vi "nx-100 (FPGA).vi"() -> ()   [LabVIEW 2019]
uses:
  <vilib>/Platform/TimedLoop/XDataNode/wakeup.ctl
  <vilib>/Platform/TimedLoop/XDataNode/XDNodeRunTimeDep.lvlib
  <vilib>/Platform/TimedLoop/XDataNode/nitl_modes.ctl
  <vilib>/Platform/TimedLoop/XDataNode/timing_clust.ctl
  <vilib>/Platform/TimedLoop/XDataNode/XDataNode.xnode
  <userlib>/_NI SPI IP/FPGA/Controllers/Public/Spi Master Inputs.ctl
  <vilib>/eio/EIONode/EIONode.xnode
  <vilib>/rvi/eio/common/nirviEmuTemplateMethod_errors.vi
  <vilib>/eio/EIOMethodNode/EIOMethodNode.xnode
  Controls/SPI Channels.ctl
  <vilib>/rvi/DataTransferAndStorage/Container/XNode/niFpgaContainer.xnode
  <vilib>/rvi/FIFO/Fifo_Resource/niFpgaFifoEmulationRefIn.vi
  <userlib>/_NI SPI IP/FPGA/Controllers/Public/Transfer Settings.ctl
  <vilib>/rvi/interface/RandomDataEmulation/nirviRandomDataFpgaReadWriteTemplate.vi
panel:
  in  "LCD Lt Timeout":i32=10000
  in  "Average?":bool
  out "Averaged Data":u16[](array[numeric])
  in  "N (# of Ave Pts 32 max)":i16
  in  "Onboard AO SPI Settings":T1={"Divide Value"=10, "Transfer Length (bits)"=32, "CS Asserted Polarity"=FALSE, "Clock Polarity (CPOL)"=TRUE, "Clock Phase (CPHA)"=FALSE, "Lengthen MISO Setup"=TRUE, "Direction Change Bit"=0, "MOSI Starts as Output"=FALSE, "Tristatable MOSI"=FALSE} {"Direction Change Bit" max=64 step=1; "Transfer Length (bits)" min=1 max=64 step=1}
  in  "Onboard AO Setpoints":fxp<+,16,3>[](array[numeric])=[0.0, 0.0, 0.0, 0.0, 0.0, 0.0, 0.0, 0.0]
  in  "Ignition Control":bool
  in  "Onboard AI Sample Divisor":u32
  in  "LCD On/Off":bool
  in  "Onboard AI Data In":u64 format="%.0x"
  out "Onboard AI":u16[](array[numeric])
  out "Onboard AI Data":u64 format="%.0x"
  in  "Onboard AI SPI Settings":T1 {"Direction Change Bit" max=64 step=1; "Transfer Length (bits)" min=1 max=64 step=1}
  in  "LCD SPI Settings":T1={"Divide Value"=9, "Transfer Length (bits)"=64, "CS Asserted Polarity"=FALSE, "Clock Polarity (CPOL)"=FALSE, "Clock Phase (CPHA)"=FALSE, "Lengthen MISO Setup"=FALSE, "Direction Change Bit"=0, "MOSI Starts as Output"=FALSE, "Tristatable MOSI"=FALSE} {"Direction Change Bit" max=64 step=1; "Transfer Length (bits)" min=1 max=64 step=1}
  in  "LCD Message":u16 format="%.0x"
  in  "LCD Send Message":bool
  out "LCD Ready For Input":bool
  in  "nx-100 Conversion Request":bool
  in  "nx-100 Manual":bool
  in  "nx-100 Trigger":bool=TRUE
  in  "nx-100 CS Mode":enum16{"All", "CS0", "CS1"}(ring)
  in  "nx-100 AI Divisor":u32
  in  "nx-100 SPI Settings":T1 {"Direction Change Bit" max=64 step=1; "Transfer Length (bits)" min=1 max=64 step=1}
  in  "nx-100 Data In":u64 format="%.0x"
  out "nx-100 AI Data":u16[](array[numeric])
  out "nx-100 Read Data":u64 format="%.0x"
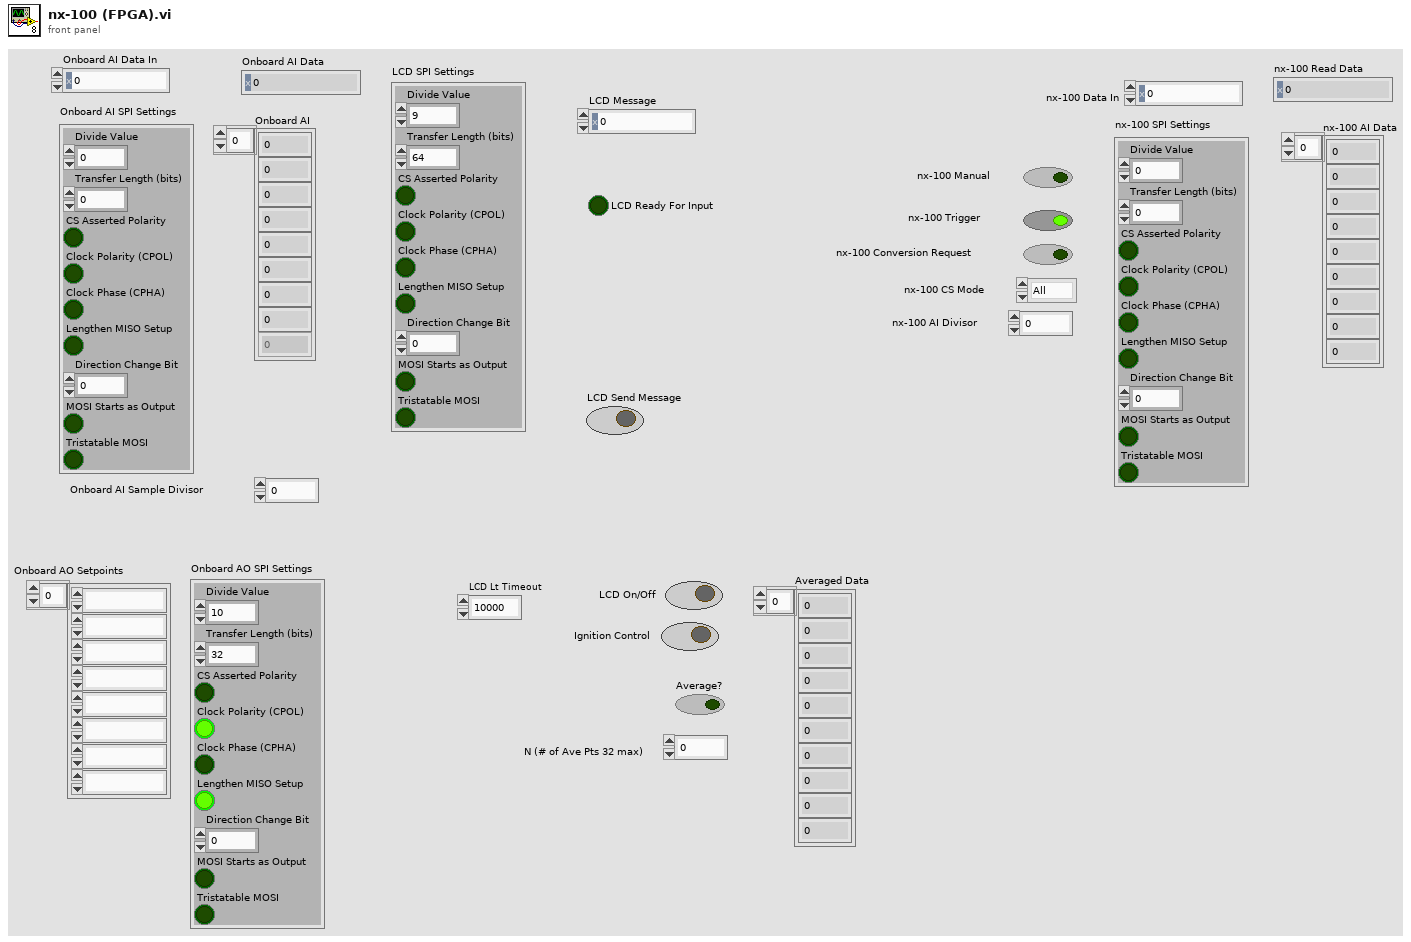
[diagram p1: front panel]
types:
  T1 = typedef "DIO SPI FPGA.lvlib/Transfer Settings.ctl" = cluster{"Divide Value":u8, "Transfer Length (bits)":u8, "CS Asserted Polarity":bool, "Clock Polarity (CPOL)":bool, "Clock Phase (CPHA)":bool, "Lengthen MISO Setup":bool, "Direction Change Bit":u8, "MOSI Starts as Output":bool, "Tristatable MOSI":bool}
  T2 = typedef "SPI Channels.ctl" = cluster{"CS":refnum<k21>, "CLK":refnum<k21>, "MOSI":refnum<k21>, "MISO":refnum<k21>}
  T3 = typedef "XDNodeRunTimeDep.lvlib/timing_clust.ctl" = cluster{"Expected End [f-1]":u64, "Actual End [f-1]":u64, "Finished Late? [f-1]":bool, "Expected End [i-1]":u64, "Actual End [i-1]":u64, "Finished Late? [i-1]":bool, "Expected Start [i]":u64, "Actual Start [i]":u64, "Expected Start [f]":u64, "Actual Start [f]":u64, "Source Name":string, "Structure Name":string, "Period":i64, "Deadline":i64, "Offset":i64, "Start":i64, "Priority":i32, "Timeout":i32, "Mode":T4, "Wakeup Reason":T5, "Error":errorcluster, "Source Type":string, "Secondary Source Type":string, "Global End Time":u64, "Global Start Time":u64, "Frame Duration":u64, "Iteration Duration":u64, "Assigned CPU":i32, "I/O Scan Engine Mode":u32}
  T4 = typedef "XDNodeRunTimeDep.lvlib/nitl_modes.ctl" = enum32{"No Change", "Process missed periods, maintain original phase", "Discard missed periods, maintain original phase", "Process missed periods, ignore original phase", "Discard missed periods, ignore original phase"}
  T5 = typedef "XDNodeRunTimeDep.lvlib/wakeup.ctl" = enum32{"Normal", "Aborted", "Asynchronous wakeup", "Timing source error", "Timed loop error", "Timeout"}
  T6 = typedef "DIO SPI FPGA.lvlib/Spi Master Inputs.ctl" = cluster{"MISO":bool}
  T7 = typedef "DIO SPI FPGA.lvlib/Spi Master Outputs.ctl" = cluster{"Chip Select":bool, "Clock":bool, "MOSI":bool, "MOSI OE":bool}
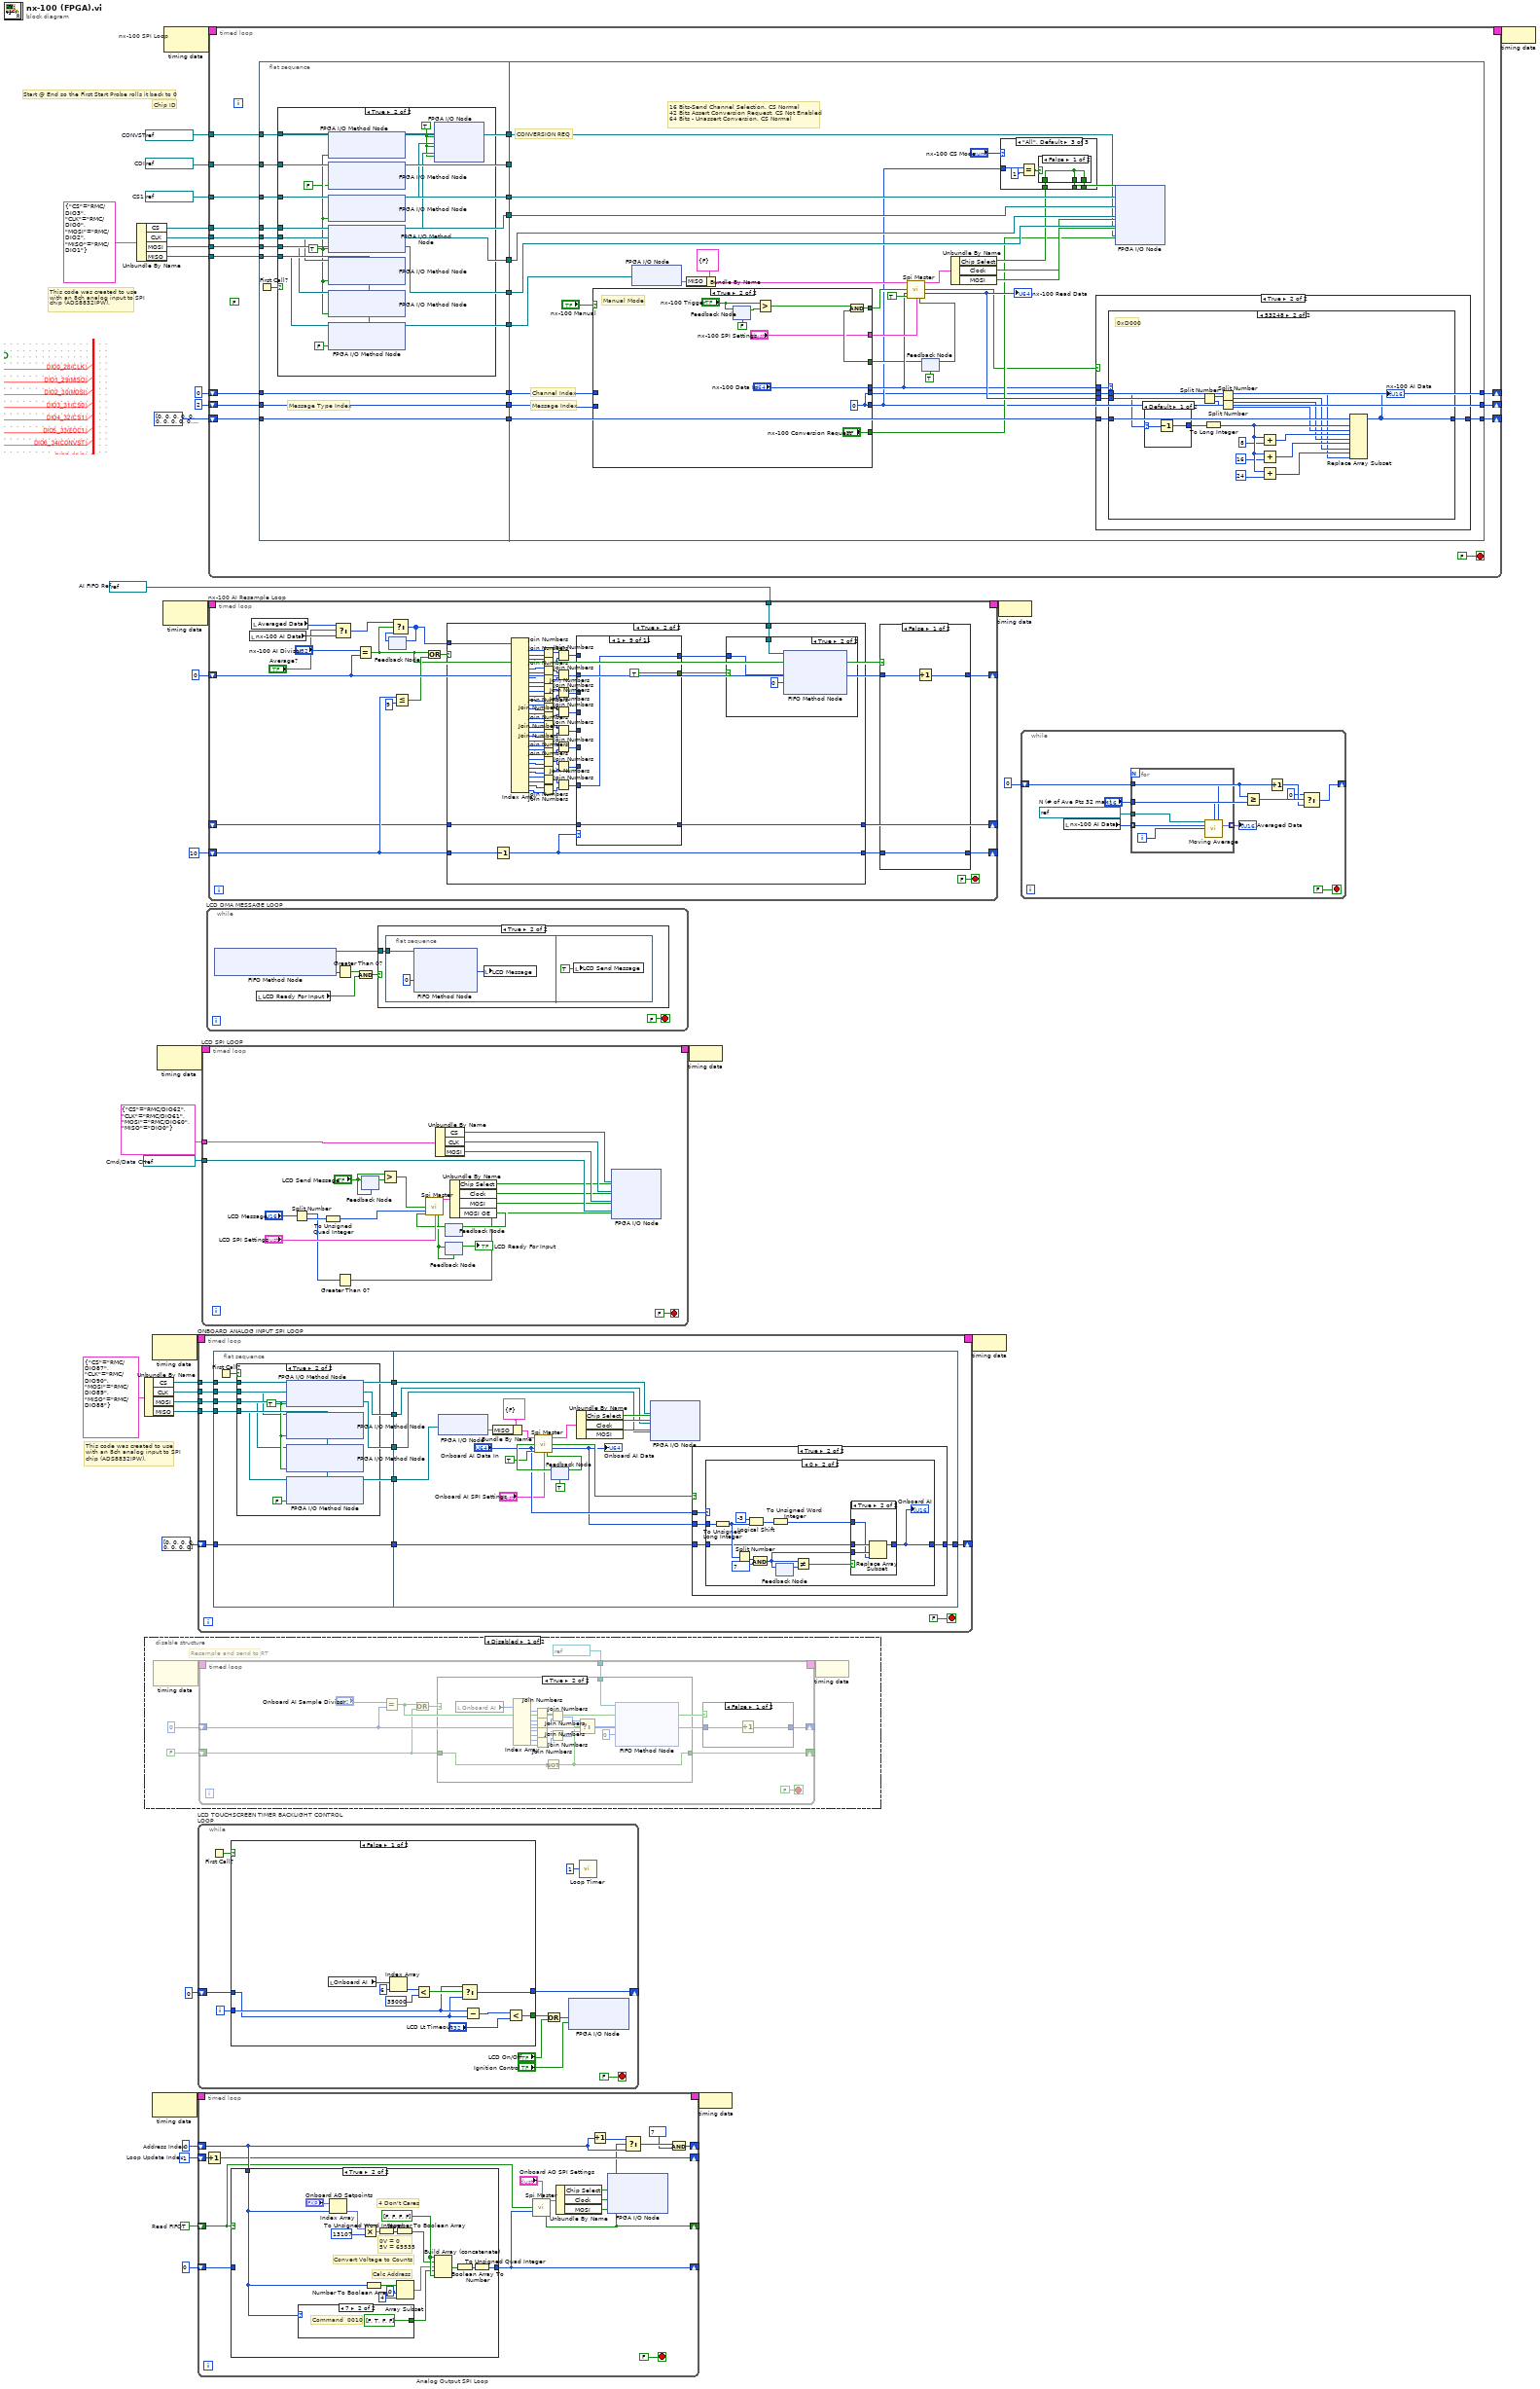
[diagram p0: block diagram]
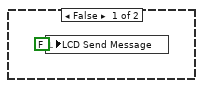
[diagram p2: hidden frame]
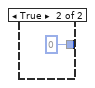
[diagram p3: hidden frame]
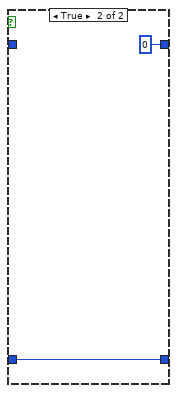
[diagram p6: hidden frame]
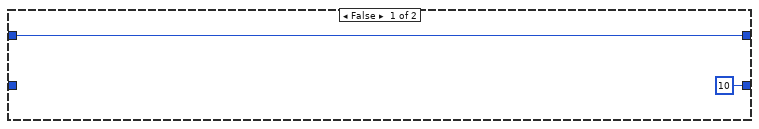
[diagram p7: hidden frame]
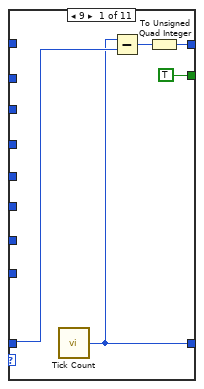
[diagram p9: hidden frame]
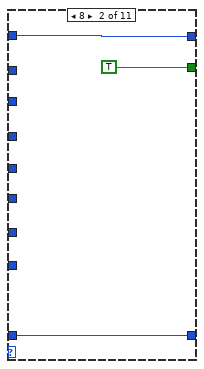
[diagram p10: hidden frame]
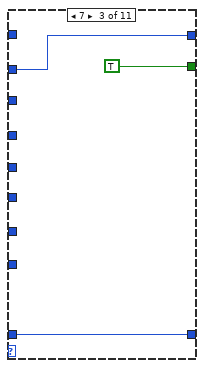
[diagram p11: hidden frame]
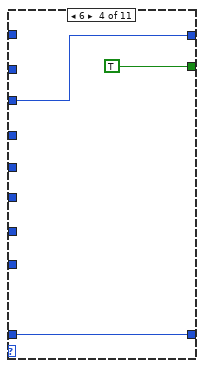
[diagram p12: hidden frame]
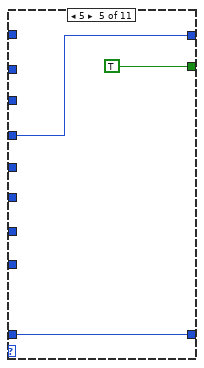
[diagram p13: hidden frame]
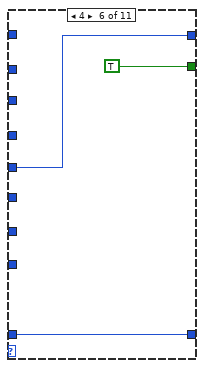
[diagram p14: hidden frame]
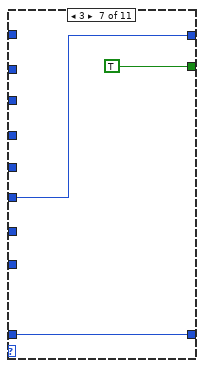
[diagram p15: hidden frame]
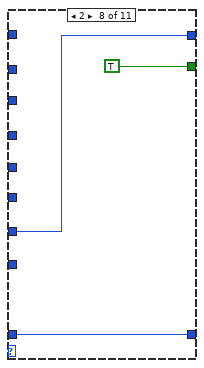
[diagram p16: hidden frame]
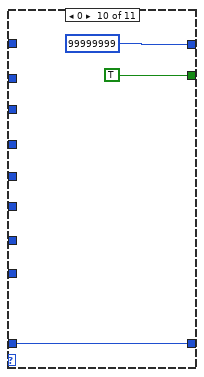
[diagram p17: hidden frame]
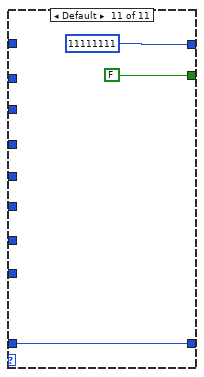
[diagram p18: hidden frame]
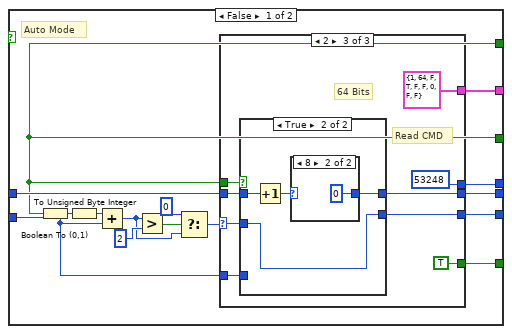
[diagram p20: hidden frame]
diagram:
  w5 = refnum<k21> "RMC/DIO63"  # Cmd/Data CH
  w19 = i16 -1  # Loop Update Index
  w20 = TRUE  # Read FIFO
  w21 = u8 0  # Address Index
  w3 = refnum<k21> "RMC/DIO6"  # CONVST
  w2 = refnum<k21> "RMC/DIO5"  # CDI
  w1 = refnum<k21> "RMC/DIO4"  # CS1
  w33 = refnum<k21> "AI Data"  # AI FIFO Ref
  # "This code was created to use\nwith an 8ch analog input to SPI\nchip (ADS8832IPW)."
  # "Start @ End so the First Start Probe rolls it back to 0"
  # "Chip ID"
  # "This code was created to use\nwith an 8ch analog input to SPI\nchip (ADS8832IPW)."
  n1 = Unbundle By Name(T2 {"CS"="RMC/DIO3", "CLK"="RMC/DIO0", "MOSI"="RMC/DIO2", "MISO"="RMC/DIO1"} ("SPI Channels")) -> ("CS"=w37:refnum<k21>, "CLK"=w36:refnum<k21>, "MOSI"=w35:refnum<k21>, "MISO"=w34:refnum<k21>)
  n2 = Unbundle By Name(T2 {"CS"="RMC/DIO87", "CLK"="RMC/DIO90", "MOSI"="RMC/DIO89", "MISO"="RMC/DIO88"} ("SPI Channels")) -> ("CS"=w29:refnum<k21>, "CLK"=w28:refnum<k21>, "MOSI"=w27:refnum<k21>, "MISO"=w26:refnum<k21>)
  n3 = disable-structure shown="Disabled" {
    frame Disabled {
      # "Resample and send to RT"
      n4 = node-c288() -> (w43:T3)  [unwired: 1 in]
      n5 = timed-loop {
        timing: w43 -> [_]
        timing-out: [_] -> w42
        shift-right: [w47] -> _
        shift-left: u32 0 ("Sample Divisor") -> [w48]
        shift-right: [w51] -> _
        shift-left: FALSE -> [w46]
        tunnel: refnum<k21> "AI Data" ("FIFO Ref") -> [w45]
        stop <- FALSE stop-if-true
        n6 = Equal?(x="Onboard AI Sample Divisor", y=w48) -> (x = y?=w49:bool)
        n7 = Or(x=w49, y=w46) -> (x .or. y?=w50:bool)
        n8 = case shown="True" w50 {
          selector: w50 -> [w56 _]
          tunnel: [w56 w60] -> w51
          tunnel: w46 -> [_ w75]
          tunnel: w45 -> [_ w57]
          frame False {
          }
          frame True {
            n9 = local read "Onboard AI"() -> (w69:u16[])
            n10 = Index Array(array=w69) -> (element #1=w58:u16, element #2=w74:u16, element #3=w73:u16, element #4=w72:u16, element #5=w66:u16, element #6=w65:u16, element #7=w64:u16, element #8=w63:u16)  [unwired: 8 in]
            n11 = Join Numbers(hi=w58, lo=w74) -> ((hi.lo)=w71:u32)
            n12 = Join Numbers(hi=w73, lo=w72) -> ((hi.lo)=w70:u32)
            n13 = Join Numbers(hi=w66, lo=w65) -> ((hi.lo)=w67:u32)
            n14 = Join Numbers(hi=w64, lo=w63) -> ((hi.lo)=w68:u32)
            n15 = Not(x=w75) -> (.not. x?=w60:bool)
            n16 = Join Numbers(hi=w71, lo=w70) -> ((hi.lo)=w62:u64)
            n17 = Join Numbers(hi=w67, lo=w68) -> ((hi.lo)=w61:u64)
            n18 = Select(t=w62, s=w60, f=w61) -> (s? t:f=w59:u64)
            n19 = xnode ("FIFO Method Node")("Element"=w59, "Timeout"=0, "FIFO In"=w57) -> ()  [unwired: 2 out]
          }
        }
        n20 = case shown="False" w49 {
          tunnel: w48 -> [w54 _]
          tunnel: [w53 u32 0] -> w47
          frame False {
            n21 = Increment(x=w54) -> (x+1=w53:u32)
          }
          frame True {
          }
        }
      }
      n22 = node-c288(w42) -> ()
    }
    frame Enabled {
    }
  }
  n23 = node-c288() -> (w32:T3)  [unwired: 1 in]
  n24 = node-c288() -> (w23:T3)  [unwired: 1 in]
  n25 = node-c288() -> (w8:T3)  [unwired: 1 in]
  n26 = node-c288() -> (w15:T3)  [unwired: 1 in]
  n27 = node-c288() -> (w17:T3)  [unwired: 1 in]
  n28 = timed-loop "ONBOARD ANALOG INPUT SPI LOOP" {
    timing: w32 -> [_]
    timing-out: [_] -> w31
    shift-right: [w89] -> _
    shift-left: u16[] [0, 0, 0, 0, 0, 0, 0, 0] -> [w90]
    tunnel: w29 -> [w88]
    tunnel: w28 -> [w87]
    tunnel: w27 -> [w86]
    tunnel: w26 -> [w85]
    stop <- FALSE stop-if-true
    n29 = flat-sequence {
      tunnel: [w97] -> w91
      tunnel: w90 -> [w97]
      tunnel: w88 -> [w96]
      tunnel: w87 -> [w95]
      tunnel: w86 -> [w94]
      tunnel: w85 -> [w93]
      tunnel: [w96] -> w84
      tunnel: [w95] -> w83
      tunnel: [w94] -> w82
      tunnel: [w93] -> w81
      tunnel: w91 -> [w112]
      tunnel: [w111] -> w89
      tunnel: w84 -> [w110]
      tunnel: w83 -> [w109]
      tunnel: w82 -> [w108]
      tunnel: w81 -> [w107]
      frame #0 {
        n30 = First Call?() -> (First Call?: T/F=w98:bool)
        n31 = case shown="True" w98 {
          tunnel: w96 -> [_ w102]
          tunnel: w95 -> [_ w101]
          tunnel: w94 -> [_ w100]
          tunnel: w93 -> [_ w99]
          frame False {
          }
          frame True {
            w104 = TRUE ("Enable")
            n32 = xnode "FPGA I/O Method Node"("FPGA I/O In"=w102, "Enable"=w104) -> ()  [unwired: 1 out]
            n33 = xnode "FPGA I/O Method Node"("FPGA I/O In"=w101, "Enable"=w104) -> ()  [unwired: 1 out]
            n34 = xnode "FPGA I/O Method Node"("FPGA I/O In"=w100, "Enable"=w104) -> ()  [unwired: 1 out]
            n35 = xnode "FPGA I/O Method Node"("FPGA I/O In"=w99, "Enable"=FALSE) -> ()  [unwired: 1 out]
          }
        }
      }
      frame #1 {
        n36 = xnode "FPGA I/O Node"("FPGA I/O In"=w107) -> ("I/O Item"=w119)  [unwired: 1 out]
        n37 = Bundle By Name(cluster=T6 {"MISO"=FALSE} ("spi input"), "MISO"=w119) -> (w120:T6)
        n38 = feedback #1(TRUE ("read data valid")) -> (w117:bool)
        n39 = call <userlib>:"Spi Master.vi"("spi input"=w120, "start strobe"=w117, "data to write"="Onboard AI Data In", "MOSI output enable done"=TRUE, "spi transfer settings"="Onboard AI SPI Settings") -> ("spi output"=w125:T7, "read data valid"=w113:bool, "read data"=w105:u64, "ready for input"=w114:bool)  [unwired: 7 in]
        "Onboard AI Data" <- w105
        n40 = feedback-in #1(w114) -> ()
        n41 = Unbundle By Name(w125) -> ("Chip Select"=w124:bool, "Clock"=w123:bool, "MOSI"=w122:bool)
        n42 = xnode "FPGA I/O Node"("I/O Item"=w124, "FPGA I/O In"=w110, "I/O Item"=w123, "FPGA I/O In"=w109, "I/O Item"=w122, "FPGA I/O In"=w108) -> ()  [unwired: 3 out]
        n43 = case shown="True" w113 {
          tunnel: "Onboard AI Data In" -> [_ w130]
          tunnel: w112 -> [w126 w129]
          tunnel: [w126 w128] -> w111
          tunnel: w105 -> [_ w127]
          frame False {
          }
          frame True {
            n44 = case shown="0" w130 {
              tunnel: w129 -> [w131 w137]
              tunnel: [w131 w136] -> w128
              tunnel: w127 -> [_ w132]
              frame Default {
              }
              frame 0 {
                n45 = To Unsigned Long Integer(number=w132) -> (unsigned 32bit integer=w138:u32)
                n46 = Split Number(x=w138) -> (lo(x)=w142:u16)  [unwired: 1 out]
                n47 = Logical Shift(y=i16 -3, x=w138) -> (x << y=w139:u32)
                n48 = And(x=w142, y=u16 7) -> (x .and. y?=w134:u16)
                n49 = To Unsigned Word Integer(number=w139) -> (unsigned 16bit integer=w133:u16)
                n50 = feedback #2() -> (w143:u16)  [unwired: 1 in]
                n51 = feedback-in #2(w134) -> ()
                n52 = Not Equal?(x=w134, y=w143) -> (x != y?=w135:bool)
                n53 = case shown="True" w135 {
                  tunnel: w137 -> [w144 w148]
                  tunnel: [w144 w147] -> w136
                  tunnel: w134 -> [_ w146]
                  tunnel: w133 -> [_ w145]
                  frame False {
                  }
                  frame True {
                    n54 = Replace Array Subset(array=w148, new element=w145, index=w146) -> (w147:u16[])
                  }
                }
                "Onboard AI" <- w136
              }
            }
          }
        }
      }
    }
  }
  n55 = timed-loop "Analog Output SPI Loop" {
    timing: w23 -> [_]
    timing-out: [_] -> w22
    shift-right: [w164] -> _
    shift-left: w20 -> [w163]
    shift-right: [w151] -> _
    shift-left: w21 -> [w167]
    shift-right: [w165] -> _
    shift-left: w19 -> [w166]
    shift-right: [w161] -> _
    shift-left: u64 0 -> [w162]
    stop <- FALSE stop-if-true
    n56 = Increment(x=w166) -> (x+1=w165:i16)
    n57 = case shown="True" w163 {
      tunnel: w167 -> [_ w170]
      tunnel: w162 -> [w168 _]
      tunnel: [w168 w172] -> w161
      frame False {
      }
      frame True {
        w183 = bool[] [FALSE, FALSE, FALSE, FALSE]
        # "4 Don't Cares"
        # "Calc Address"
        # "0V = 0\n5V = 65535"
        # "Convert Voltage to Counts"
        n58 = case shown="7" w170 {
          tunnel: [bool[] [FALSE, FALSE, FALSE, FALSE] bool[] [FALSE, TRUE, FALSE, FALSE]] -> w182
          frame Default {
            # "Command  0000"
          }
          frame 7 {
            # "Command  0010"
          }
        }
        n59 = Index Array(array="Onboard AO Setpoints", index=w170) -> (element=w169:fxp<+,16,3>)
        n60 = Multiply(x=w169, y=u16 13107 ("-x")) -> (x*y=w173:fxp<+,32,19>)
        n61 = Number To Boolean Array(number=w170) -> (Boolean array=w175:bool[])
        n62 = To Unsigned Word Integer(number=w173) -> (unsigned 16bit integer=w178:u16)
        n63 = Number To Boolean Array(number=w178) -> (Boolean array=w180:bool[])
        n64 = Array Subset(array=w175, index=0, length=4) -> (w181:bool[])
        n65 = Build Array (concatenate)(w183, w180, w181, w182, w183) -> (w184:bool[])
        n66 = Boolean Array To Number(Boolean array=w184) -> (number=w179:u32)
        n67 = To Unsigned Quad Integer(1:w179) -> (0:w172:u64)
      }
    }
    n68 = call <userlib>:"Spi Master.vi"("start strobe"=w163, "data to write"=w161, "spi transfer settings"="Onboard AO SPI Settings") -> ("spi output"=w155:T7, "ready for input"=w164:bool)  [unwired: 9 in, 2 out]
    n69 = Unbundle By Name(w155) -> ("Chip Select"=w156:bool, "Clock"=w157:bool, "MOSI"=w158:bool)
    n70 = Increment(x=w167) -> (x+1=w159:u8)
    n71 = xnode "FPGA I/O Node"("RMC/DIO91"=w156, "RMC/DIO92"=w157, "RMC/DIO93"=w158) -> ()  [unwired: 3 in, 3 out]
    n72 = Select(t=w159, s=w164, f=w167) -> (s? t:f=w153:u8)
    n73 = And(x=w153, y=u8 7) -> (x .and. y?=w151:u8)
  }
  n74 = while "LCD TOUCHSCREEN TIMER BACKLIGHT CONTROL LOOP" {
    shift-right: [w194] -> _
    shift-left: 0 -> [w195]
    i -> [w193]
    stop <- FALSE stop-if-true
    n75 = First Call?() -> (First Call?: T/F=w197:bool)
    n76 = case shown="False" w197 {
      tunnel: w195 -> [w199 _]
      tunnel: [w201 w211] -> w194
      tunnel: w193 -> [w200 w211]
      tunnel: [w202 TRUE] -> w192
      frame False {
        n77 = local read "Onboard AI"() -> (w209:u16[])
        n78 = Index Array(array=w209, index=6) -> (element=w207:u16)
        n79 = Less?(x=w207, y=u16 35000 ("LCD Threshold")) -> (x < y?=w203:bool)
        n80 = Select(t=w200, s=w203, f=w199) -> (s? t:f=w201:i32)
        n81 = Subtract(x=w200, y=w199) -> (x-y=w205:i32)
        n82 = Less?(x=w205, y="LCD Lt Timeout") -> (x < y?=w202:bool)
      }
      frame True {
        w212 = FALSE ("DIO64 Out?")
        w215 = TRUE ("DIO65 Out?")
        w214 = FALSE ("DIO64 Out?")
        n83 = xnode "FPGA I/O Method Node"("FPGA I/O In"=refnum<k21> "RMC/DIO64" ("FPGA I/O"), "Enable"=w214) -> ("FPGA I/O Out"=w217:refnum<k21>)
        n84 = xnode "FPGA I/O Method Node"("FPGA I/O In"=refnum<k21> "RMC/DIO65" ("FPGA I/O"), "Enable"=w215) -> ("FPGA I/O Out"=w218:refnum<k21>)
        n85 = xnode "FPGA I/O Method Node"("FPGA I/O In"=refnum<k21> "RMC/DIO66" ("FPGA I/O"), "Enable"=w215) -> ("FPGA I/O Out"=w221:refnum<k21>)
        n86 = xnode "FPGA I/O Method Node"("FPGA I/O In"=refnum<k21> "RMC/DIO67" ("FPGA I/O"), "Enable"=w214) -> ("FPGA I/O Out"=w222:refnum<k21>)
        n87 = xnode "FPGA I/O Method Node"("FPGA I/O In"=w217, "Data"=w212) -> ()  [unwired: 1 out]
        n88 = xnode "FPGA I/O Method Node"("FPGA I/O In"=w218, "Data"=TRUE) -> ()  [unwired: 1 out]
        n89 = xnode "FPGA I/O Method Node"("FPGA I/O In"=w221, "Data"=w212) -> ()  [unwired: 1 out]
        n90 = xnode "FPGA I/O Method Node"("FPGA I/O In"=w222, "Data"=w212) -> ()  [unwired: 1 out]
      }
    }
    n91 = Or(x=w192, y="LCD On/Off") -> (x .or. y?=w191:bool)
    n92 = xnode "FPGA I/O Node"("RMC/DIO68"=w191, "RMC/DIO80"="Ignition Control") -> ()  [unwired: 2 in, 2 out]
    n93 = call "Loop Timer"("Count(mSec)"=u32 1 ("Count(Ticks)")) -> ()  [unwired: 1 out]
  }
  n94 = timed-loop "LCD SPI LOOP" {
    timing: w8 -> [_]
    timing-out: [_] -> w7
    tunnel: T2 {"CS"="RMC/DIO62", "CLK"="RMC/DIO61", "MOSI"="RMC/DIO60", "MISO"="DIO0"} ("SPI Channels") -> [w245]
    tunnel: w5 -> [w244]
    stop <- FALSE stop-if-true
    n95 = Split Number(x="LCD Message") -> (hi(x)=w225:u8, lo(x)=w227:u8)
    n96 = To Unsigned Quad Integer(1:w227) -> (0:w226:u64)
    n97 = Greater Than 0?(x=w225) -> (x > 0?=w224:bool)
    n98 = feedback #3("LCD Send Message") -> (w233:bool)
    n99 = feedback-in #3("LCD Send Message") -> ()
    n100 = Greater?(x="LCD Send Message", y=w233) -> (0:w232:bool)
    n101 = Unbundle By Name(w245) -> ("CS"=w240:refnum<k21>, "CLK"=w239:refnum<k21>, "MOSI"=w238:refnum<k21>)
    n102 = feedback #4() -> (w236:bool)  [unwired: 1 in]
    n103 = call <userlib>:"Spi Master.vi"("start strobe"=w232, "data to write"=w226, "MOSI output enable done"=w236, "spi transfer settings"="LCD SPI Settings") -> ("spi output"=w243:T7, "ready for input"=w230:bool)  [unwired: 8 in, 2 out]
    n104 = feedback #5(w230) -> (→"LCD Ready For Input":bool)
    n105 = feedback-in #5(w230) -> ()
    n106 = Unbundle By Name(w243) -> ("Chip Select"=w234:bool, "Clock"=w235:bool, "MOSI"=w237:bool, "MOSI OE"=w241:bool)
    n107 = feedback-in #4(w241) -> ()
    n108 = xnode "FPGA I/O Node"("I/O Item"=w234, "FPGA I/O In"=w240, "I/O Item"=w235, "FPGA I/O In"=w239, "I/O Item"=w237, "FPGA I/O In"=w238, "I/O Item"=w224, "FPGA I/O In"=w244) -> ()  [unwired: 4 out]
  }
  n109 = while "LCD DMA MESSAGE LOOP" {
    stop <- FALSE stop-if-true
    n110 = xnode ("FIFO Method Node")() -> ("Number of Elements to Read"=w250:u32, "FIFO Out"=w253:refnum<k21>)  [unwired: 1 in]
    n111 = local read "LCD Ready For Input"() -> (w251:bool)
    n112 = Greater Than 0?(x=w250) -> (x > 0?=w249:bool)
    n113 = And(x=w249, y=w251) -> (x .and. y?=w252:bool)
    n114 = case shown="True" w252 {
      tunnel: w253 -> [_ w256]
      frame False {
        n115 = local write "LCD Send Message"(FALSE ("Send Message")) -> ()
      }
      frame True {
        n116 = flat-sequence {
          tunnel: w256 -> [w257]
          frame #0 {
            n117 = xnode ("FIFO Method Node")("Timeout"=0, "FIFO In"=w257) -> ("Element"=w258:u64)  [unwired: 2 out]
            n118 = local write "LCD Message"(w258) -> ()
          }
          frame #1 {
            n119 = local write "LCD Send Message"(TRUE ("Send Message")) -> ()
          }
        }
      }
    }
  }
  n120 = timed-loop "nx-100 AI Resample Loop" {
    timing: w15 -> [_]
    timing-out: [_] -> w14
    shift-right: [w278] -> _
    shift-left: u32 0 ("Sample Divisor") -> [w279]
    shift-right: [w275] -> _
    shift-left: u32 10 ("Sample Divisor") -> [w276]
    tunnel: w33 -> [w277]
    shift-right: [w267] -> _
    shift-left: _ -> [w266]
    stop <- FALSE stop-if-true
    n121 = local read "nx-100 AI Data"() -> (w263:u16[])
    n122 = local read "Averaged Data"() -> (w264:u16[])
    n123 = Select(t=w264, s="Average?", f=w263) -> (s? t:f=w261:u16[])
    n124 = Equal?(x="nx-100 AI Divisor", y=w279) -> (x = y?=w269:bool)
    n125 = feedback #6() -> (w268:u16[])  [unwired: 1 in]
    n126 = Select(t=w261, s=w269, f=w268) -> (s? t:f=w265:u16[])
    n127 = feedback-in #6(w265) -> ()
    n128 = Less Or Equal?(x=w276, y=u32 9) -> (x <= y?=w271:bool)
    n129 = Or(x=w269, y=w271) -> (x .or. y?=w274:bool)
    n130 = case shown="True" w274 {
      tunnel: w277 -> [_ w340]
      tunnel: w276 -> [_ w322]
      tunnel: [u32 10 w290] -> w270
      tunnel: w265 -> [_ w292]
      tunnel: [w286 w289] -> w267
      tunnel: w266 -> [w286 w288]
      frame False {
      }
      frame True {
        n131 = Decrement(x=w322) -> (x-1=w290:u32)
        n132 = Index Array(array=w292) -> (element #1=w341:u16, element #2=w351:u16, element #3=w350:u16, element #4=w349:u16, element #5=w345:u16, element #6=w344:u16, element #7=w343:u16, element #8=w342:u16, element #9=w335:u16, element #10=w334:u16, element #11=w333:u16, element #12=w332:u16, element #13=w331:u16, element #14=w330:u16, element #15=w329:u16, element #16=w328:u16, element #17=w315:u16, element #18=w314:u16, element #19=w313:u16, element #20=w312:u16, element #21=w309:u16, element #22=w308:u16, element #23=w307:u16, element #24=w306:u16, element #25=w305:u16, element #26=w304:u16, element #27=w303:u16, element #28=w302:u16, element #29=w301:u16, element #30=w300:u16, element #31=w299:u16, element #32=w298:u16)  [unwired: 32 in]
        n133 = Join Numbers(hi=w341, lo=w351) -> ((hi.lo)=w348:u32)
        n134 = Join Numbers(hi=w350, lo=w349) -> ((hi.lo)=w347:u32)
        n135 = Join Numbers(hi=w345, lo=w344) -> ((hi.lo)=w293:u32)
        n136 = Join Numbers(hi=w343, lo=w342) -> ((hi.lo)=w346:u32)
        n137 = Join Numbers(hi=w335, lo=w334) -> ((hi.lo)=w336:u32)
        n138 = Join Numbers(hi=w333, lo=w332) -> ((hi.lo)=w337:u32)
        n139 = Join Numbers(hi=w331, lo=w330) -> ((hi.lo)=w339:u32)
        n140 = Join Numbers(hi=w329, lo=w328) -> ((hi.lo)=w338:u32)
        n141 = Join Numbers(hi=w315, lo=w314) -> ((hi.lo)=w320:u32)
        n142 = Join Numbers(hi=w313, lo=w312) -> ((hi.lo)=w321:u32)
        n143 = Join Numbers(hi=w309, lo=w308) -> ((hi.lo)=w316:u32)
        n144 = Join Numbers(hi=w307, lo=w306) -> ((hi.lo)=w317:u32)
        n145 = Join Numbers(hi=w305, lo=w304) -> ((hi.lo)=w319:u32)
        n146 = Join Numbers(hi=w303, lo=w302) -> ((hi.lo)=w318:u32)
        n147 = Join Numbers(hi=w301, lo=w300) -> ((hi.lo)=w310:u32)
        n148 = Join Numbers(hi=w299, lo=w298) -> ((hi.lo)=w311:u32)
        n149 = Join Numbers(hi=w348, lo=w347) -> ((hi.lo)=w327:u64)
        n150 = Join Numbers(hi=w293, lo=w346) -> ((hi.lo)=w326:u64)
        n151 = Join Numbers(hi=w336, lo=w337) -> ((hi.lo)=w325:u64)
        n152 = Join Numbers(hi=w339, lo=w338) -> ((hi.lo)=w324:u64)
        n153 = Join Numbers(hi=w320, lo=w321) -> ((hi.lo)=w297:u64)
        n154 = Join Numbers(hi=w316, lo=w317) -> ((hi.lo)=w296:u64)
        n155 = Join Numbers(hi=w319, lo=w318) -> ((hi.lo)=w295:u64)
        n156 = Join Numbers(hi=w310, lo=w311) -> ((hi.lo)=w294:u64)
        n157 = case shown="1" w290 {
          tunnel: w327 -> [_ w362 _ _ _ _ _ _ _ _ _]
          tunnel: w326 -> [_ _ w365 _ _ _ _ _ _ _ _]
          tunnel: w325 -> [_ _ _ w368 _ _ _ _ _ _ _]
          tunnel: w324 -> [_ _ _ _ w371 _ _ _ _ _ _]
          tunnel: [w356 w362 w365 w368 w371 w374 w377 w380 w383 u64 99999999 u64 11111111] -> w323
          tunnel: w297 -> [_ _ _ _ _ w374 _ _ _ _ _]
          tunnel: w296 -> [_ _ _ _ _ _ w377 _ _ _ _]
          tunnel: w295 -> [_ _ _ _ _ _ _ w380 _ _ _]
          tunnel: w294 -> [_ _ _ _ _ _ _ _ w383 _ _]
          tunnel: [TRUE TRUE TRUE TRUE TRUE TRUE TRUE TRUE TRUE TRUE FALSE] -> w291
          tunnel: [w355 w360 w363 w366 w369 w372 w375 w378 w381 w384 w387] -> w289
          tunnel: w288 -> [w358 w360 w363 w366 w369 w372 w375 w378 w381 w384 w387]
          frame 9 {
            n158 = call "Tick Count"() -> ("Tick Count(uSec)"=w355:u32)
            n159 = Subtract(x=w355, y=w358) -> (x-y=w357:u32)
            n160 = To Unsigned Quad Integer(1:w357) -> (0:w356:u64)
          }
          frame 8 {
          }
          frame 7 {
          }
          frame 6 {
          }
          frame 5 {
          }
          frame 4 {
          }
          frame 3 {
          }
          frame 2 {
          }
          frame 1 {
          }
          frame 0 {
          }
          frame Default {
          }
        }
        n161 = case shown="True" w291 {
          tunnel: w340 -> [_ w353]
          tunnel: w323 -> [_ w352]
          frame False {
          }
          frame True {
            n162 = xnode ("FIFO Method Node")("Element"=w352, "Timeout"=0, "FIFO In"=w353) -> ()  [unwired: 2 out]
          }
        }
      }
    }
    n163 = case shown="False" w269 {
      tunnel: w279 -> [w283 _]
      tunnel: [w282 u32 0] -> w278
      tunnel: w270 -> [w281 w284]
      tunnel: [w281 w284] -> w275
      frame False {
        n164 = Increment(x=w283) -> (x+1=w282:u32)
      }
      frame True {
      }
    }
  }
  n165 = timed-loop "nx-100 SPI Loop" {
    shift-right: [w413] -> _
    shift-left: u16[] [0, 0, 0, 0, 0, 0, 0, 0, 0, 0, 0, 0, 0, 0, 0, 0, 0, 0, 0, 0, 0, 0, 0, 0, 0, 0, 0, 0, 0, 0, 0, 0] -> [w414]
    tunnel: w37 -> [w412]
    tunnel: w36 -> [w411]
    tunnel: w35 -> [w410]
    tunnel: w34 -> [w409]
    tunnel: w1 -> [w408]
    tunnel: w3 -> [w407]
    tunnel: w2 -> [w406]
    timing: w17 -> [_]
    timing-out: [_] -> w16
    shift-right: [w395] -> _
    shift-left: u8 2 ("lo(x)") -> [w396]
    shift-right: [w392] -> _
    shift-left: u8 0 ("lo(x)") -> [w393]
    stop <- FALSE stop-if-true
    (unwired) FALSE ("Enable")
    n166 = flat-sequence {
      tunnel: [w425] -> w405
      tunnel: w414 -> [w425]
      tunnel: w412 -> [w424]
      tunnel: w411 -> [w423]
      tunnel: w410 -> [w422]
      tunnel: w409 -> [w421]
      tunnel: [w424] -> w404
      tunnel: [w423] -> w403
      tunnel: [w422] -> w402
      tunnel: [w421] -> w401
      tunnel: w408 -> [w420]
      tunnel: w407 -> [w419]
      tunnel: w406 -> [w418]
      tunnel: [w420] -> w400
      tunnel: [w418] -> w399
      tunnel: [w419] -> w398
      tunnel: [w417] -> w397
      tunnel: w396 -> [w417]
      tunnel: [w416] -> w394
      tunnel: w393 -> [w416]
      tunnel: w405 -> [w468]
      tunnel: [w467] -> w413
      tunnel: w404 -> [w463]
      tunnel: w403 -> [w466]
      tunnel: w402 -> [w465]
      tunnel: w401 -> [w464]
      tunnel: w400 -> [w462]
      tunnel: w399 -> [_]
      tunnel: w398 -> [w448]
      tunnel: w397 -> [w449]
      tunnel: [w443] -> w395
      tunnel: w394 -> [w442]
      tunnel: [w441] -> w392
      frame #0 {
        # "Message Type Index"
        n167 = First Call?() -> (First Call?: T/F=w426:bool)
        n168 = case shown="True" w426 {
          tunnel: w424 -> [_ w439]
          tunnel: w423 -> [_ w438]
          tunnel: w422 -> [_ w437]
          tunnel: w421 -> [_ w436]
          tunnel: w420 -> [_ w435]
          tunnel: w419 -> [_ w434]
          tunnel: w418 -> [_ w432]
          frame False {
          }
          frame True {
            w427 = TRUE ("I/O Item")
            w433 = TRUE ("Enable")
            n169 = xnode "FPGA I/O Method Node"("FPGA I/O In"=w434, "Enable"=w433) -> ("FPGA I/O Out"=w428:refnum<k21>)
            n170 = xnode "FPGA I/O Method Node"("FPGA I/O In"=w432, "Enable"=FALSE) -> ()  [unwired: 1 out]
            n171 = xnode "FPGA I/O Method Node"("FPGA I/O In"=w435, "Enable"=w433) -> ("FPGA I/O Out"=w431:refnum<k21>)
            n172 = xnode "FPGA I/O Method Node"("FPGA I/O In"=w439, "Enable"=w433) -> ("FPGA I/O Out"=w430:refnum<k21>)
            n173 = xnode "FPGA I/O Method Node"("FPGA I/O In"=w438, "Enable"=w433) -> ()  [unwired: 1 out]
            n174 = xnode "FPGA I/O Method Node"("FPGA I/O In"=w437, "Enable"=w433) -> ()  [unwired: 1 out]
            n175 = xnode "FPGA I/O Method Node"("FPGA I/O In"=w436, "Enable"=FALSE) -> ()  [unwired: 1 out]
            n176 = xnode "FPGA I/O Node"("I/O Item"=w427, "FPGA I/O In"=w428, "I/O Item"=w427, "FPGA I/O In"=w431, "I/O Item"=w427, "FPGA I/O In"=w430) -> ()  [unwired: 3 out]
          }
        }
      }
      frame #1 {
        # "Message Index"
        # "Channel Index"
        # "16 Bits-Send Channel Selection, CS Normal \n42 Bits Assert Conversion Request, CS Not Enabled\n64 Bits - Unassert Conversion, CS Normal"
        # "CONVERSION REQ"
        n177 = xnode "FPGA I/O Node"("FPGA I/O In"=w464) -> ("I/O Item"=w469)  [unwired: 1 out]
        n178 = Bundle By Name(cluster=T6 {"MISO"=FALSE} ("spi input"), "MISO"=w469) -> (w470:T6)
        n179 = feedback #7(TRUE ("Chip Select")) -> (w445:bool)
        n180 = case shown="True" "nx-100 Manual" {
          tunnel: w445 -> [w476 w523]
          tunnel: [w476 w522] -> w451
          tunnel: [w481 "nx-100 SPI Settings"] -> w450
          tunnel: w449 -> [w475 _]
          tunnel: [w477 "nx-100 Data In"] -> w446
          tunnel: [w474 w518] -> w443
          tunnel: [w480 "nx-100 Conversion Request"] -> w447
          tunnel: w442 -> [w479 _]
          tunnel: [w478 w518] -> w441
          frame False {
            # "Auto Mode"
            n181 = Boolean To (0,1)(Boolean=w476) -> (0, 1=w488:i16)
            n182 = To Unsigned Byte Integer(number=w488) -> (unsigned 8bit integer=w487:u8)
            n183 = Add(x=w487, y=w475) -> (x+y=w483:u8)
            n184 = Greater?(x=w483, y=u8 2) -> (0:w485:bool)
            n185 = Select(t=u8 0 ("y"), s=w485, f=w483) -> (s? t:f=w482:u8)
            n186 = case shown="2" w482 {
              selector: w482 -> [w492 w496 w504]
              tunnel: [T1 {"Divide Value"=1, "Transfer Length (bits)"=16, "CS Asserted Polarity"=FALSE, "Clock Polarity (CPOL)"=TRUE, "Clock Phase (CPHA)"=FALSE, "Lengthen MISO Setup"=FALSE, "Direction Change Bit"=0, "MOSI Starts as Output"=FALSE, "Tristatable MOSI"=FALSE} ("Master Settings 2") T1 {"Divide Value"=1, "Transfer Length (bits)"=42, "CS Asserted Polarity"=FALSE, "Clock Polarity (CPOL)"=TRUE, "Clock Phase (CPHA)"=FALSE, "Lengthen MISO Setup"=FALSE, "Direction Change Bit"=0, "MOSI Starts as Output"=FALSE, "Tristatable MOSI"=FALSE} ("Master Settings 2") T1 {"Divide Value"=1, "Transfer Length (bits)"=64, "CS Asserted Polarity"=FALSE, "Clock Polarity (CPOL)"=TRUE, "Clock Phase (CPHA)"=FALSE, "Lengthen MISO Setup"=FALSE, "Direction Change Bit"=0, "MOSI Starts as Output"=FALSE, "Tristatable MOSI"=FALSE} ("Master Settings 2")] -> w481
              tunnel: [TRUE ("I/O Item") FALSE ("I/O Item") TRUE ("I/O Item")] -> w480
              tunnel: w479 -> [w491 w497 w503]
              tunnel: [w491 w497 w502] -> w478
              tunnel: [w489 u64 0 u64 53248] -> w477
              tunnel: w476 -> [_ _ w506]
              tunnel: w475 -> [_ _ w501]
              tunnel: [w492 w496 w505] -> w474
              frame 0, Default {
                # "16 Bits"
                # "Channel Select"
                # "0x#000"
                n187 = To Unsigned Quad Integer(1:w491) -> (0:w490:u64)
                n188 = Logical Shift(y=i16 12, x=w490) -> (x << y=w489:u64)
              }
              frame 1 {
                # "Conversion Request Asserted"
                # "42 Bits"
                # "Dont Care"
              }
              frame 2 {
                # "64 Bits"
                # "Read CMD"
                n189 = case shown="True" w506 {
                  tunnel: [w510 w514] -> w505
                  tunnel: w504 -> [_ w514]
                  tunnel: w503 -> [w511 w515]
                  tunnel: [w511 w512] -> w502
                  tunnel: w501 -> [w510 _]
                  frame False {
                  }
                  frame True {
                    n190 = Increment(x=w515) -> (x+1=w513:u8)
                    n191 = case shown="8" w513 {
                      selector: w513 -> [w516 _]
                      tunnel: [w516 u8 0] -> w512
                      frame Default {
                      }
                      frame 8 {
                      }
                    }
                  }
                }
              }
            }
          }
          frame True {
            w518 = u8 0 ("y")
            # "Manual Mode"
            n192 = feedback #8(FALSE) -> (w527:bool)
            n193 = feedback-in #8("nx-100 Trigger") -> ()
            n194 = Greater?(x="nx-100 Trigger", y=w527) -> (0:w524:bool)
            n195 = And(x=w524, y=w523) -> (x .and. y?=w522:bool)
          }
        }
        n196 = call <userlib>:"Spi Master.vi"("spi input"=w470, "start strobe"=w451, "data to write"=w446, "MOSI output enable done"=TRUE, "spi transfer settings"=w450) -> ("spi output"=w473:T7, "read data valid"=w444:bool, "read data"=w458:u64, "ready for input"=w460:bool)  [unwired: 7 in]
        "nx-100 Read Data" <- w458
        n197 = feedback-in #7(w460) -> ()
        n198 = Unbundle By Name(w473) -> ("Chip Select"=w455:bool, "Clock"=w459:bool, "MOSI"=w472:bool)
        n199 = case shown="\"All\", Default" "nx-100 CS Mode" {
          tunnel: w455 -> [w529 w531 w535]
          tunnel: [TRUE ("Chip Select") w531 w534] -> w454
          tunnel: [w529 TRUE ("Chip Select") w533] -> w453
          tunnel: w443 -> [_ _ w537]
          frame "CS1" {
          }
          frame "CS0" {
          }
          frame "All", Default {
            n200 = Equal?(x=w537, y=u8 1) -> (x = y?=w532:bool)
            n201 = case shown="False" w532 {
              tunnel: w535 -> [w538 _]
              tunnel: [w538 w539] -> w534
              tunnel: [w538 w539] -> w533
              frame False {
              }
              frame True {
                w539 = TRUE ("Chip Select")
              }
            }
          }
        }
        n202 = case shown="True" w444 {
          tunnel: w458 -> [_ w545]
          tunnel: w468 -> [w540 w544]
          tunnel: [w540 w543] -> w467
          tunnel: w446 -> [_ w542]
          tunnel: w441 -> [_ w541]
          frame False {
          }
          frame True {
            n203 = case shown="53248" w542 {
              tunnel: w545 -> [_ w564]
              tunnel: w544 -> [w546 w562]
              tunnel: [w546 w563] -> w543
              tunnel: w541 -> [_ w547]
              frame Default {
              }
              frame 53248 {
                # "0xD000"
                n204 = case shown="Default" w547 {
                  selector: w547 -> [w565 _]
                  tunnel: [w566 u8 7] -> w548
                  frame Default {
                    n205 = Decrement(x=w565) -> (x-1=w566:u8)
                  }
                  frame 0 {
                  }
                }
                n206 = Split Number(x=w564) -> (hi(x)=w561:u32, lo(x)=w560:u32)
                n207 = To Long Integer(number=w548) -> (32bit integer=w559:i32)
                n208 = Split Number(x=w561) -> (hi(x)=w551:u16, lo(x)=w552:u16)
                n209 = Split Number(x=w560) -> (hi(x)=w553:u16, lo(x)=w554:u16)
                n210 = Add(x=w559, y=8) -> (x+y=w557:i32)
                n211 = Add(x=w559, y=16) -> (x+y=w556:i32)
                n212 = Add(x=w559, y=24) -> (x+y=w555:i32)
                n213 = Replace Array Subset(array=w562, new element #1=w554, index #1=w559, new element #2=w553, index #2=w557, new element #3=w552, index #3=w556, new element #4=w551, index #4=w555) -> (w563:u16[])
                "nx-100 AI Data" <- w563
              }
            }
          }
        }
        n214 = xnode "FPGA I/O Node"("I/O Item"=w453, "FPGA I/O In"=w462, "I/O Item"=w454, "FPGA I/O In"=w463, "I/O Item"=w459, "FPGA I/O In"=w466, "I/O Item"=w472, "FPGA I/O In"=w465, "I/O Item"=w447, "FPGA I/O In"=w448) -> ()  [unwired: 5 out]
      }
    }
  }
  n215 = node-c288(w7) -> ()
  n216 = node-c288(w22) -> ()
  n217 = node-c288(w31) -> ()
  n218 = node-c288(w14) -> ()
  n219 = while {
    shift-right: [w573] -> _
    shift-left: i16 0 ("Moving Point Index") -> [w578]
    stop <- FALSE stop-if-true
    n220 = local read "nx-100 AI Data"() -> (w579:u16[])
    n221 = for {
      tunnel: w579 -> [w585] mode=indexing
      tunnel: w578 -> [w582]
      tunnel: "N (# of Ave Pts 32 max)" -> [w583]
      tunnel: [w581] -> w571 mode=indexing
      tunnel: refnum<k21> "nx-100 Average Buffer" ("Memory In") -> [w580]
      i -> [w584]
      n222 = call "Moving Average.vi"("Memory In"=w580, "N (# of Ave Pts 127 max)"=w583, "Moving Point Index"=w582, "Data IN"=w585, "Channel#"=w584) -> ("Averaged Data"=w581:fxp<+/-,28,17>)  [unwired: 10 in]
    }
    "Averaged Data" <- w571
    n223 = Greater Or Equal?(x=w578, y="N (# of Ave Pts 32 max)") -> (x >= y?=w576:bool)
    n224 = Increment(x=w578) -> (x+1=w575:i16)
    n225 = Select(t=i16 0, s=w576, f=w575) -> (s? t:f=w573:i16)
  }
  n226 = node-c288(w16) -> ()
